vi "GUI.vi"(8 "error in (no error)":errorcluster) -> (0 "error out":errorcluster)   [LabVIEW 2020]
uses:
  CTLs/playback status.ctl
  FGVs/FGVstates.ctl
  CTLs/GUI_states.ctl
  CTLs/ButtonRefs.ctl
  FGVs/AppStates.ctl
panel:
  in  "Skip Forward Button":bool
  in  "Skip Back Button":bool
  out "Playback status":T1
  in  "Playlist":i32(listbox)
  out "Right Channel":dbl[](graph)
  out "Left Channel":dbl[](graph)
  in  "Pause Button":bool
  in  "Stop Button":bool
  in  "Play Button":bool
  in  "Playback Timeline":i32(slide) scale=0.0..11305728.0
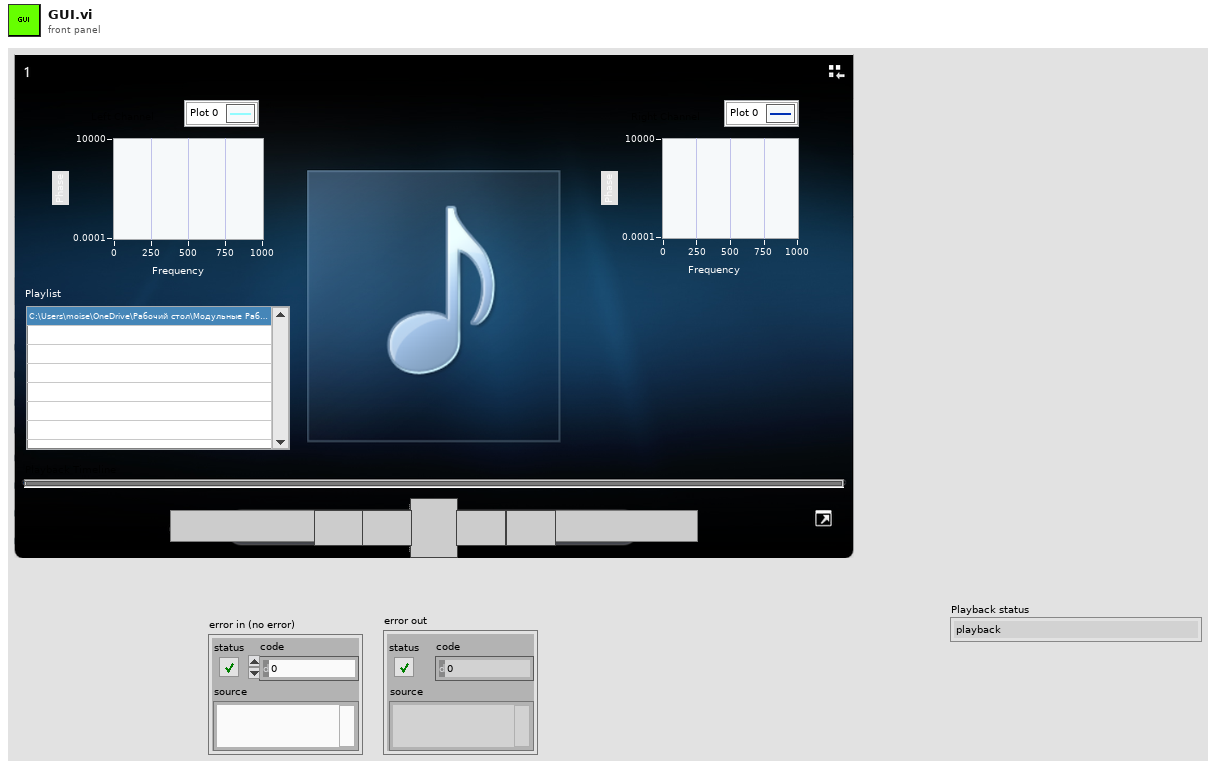
[diagram p1: front panel]
types:
  T1 = typedef "playback status.ctl" = enum16{"playback", "pause", "stop"}
  T2 = typedef "ButtonRefs.ctl" = cluster{"Button_play":refnum<vi>, "Button_pause":refnum<vi>, "Button_stop":refnum<vi>, "Playlist":refnum<vi>, "Playback status":refnum<vi>, "Playback Timeline":refnum<vi>, "Right Channel":refnum<vi>, "Left Channel":refnum<vi>, "Skip Forward Button":refnum<vi>, "Skip Back Button":refnum<vi>}
  T3 = typedef "GUI_states.ctl" = enum16{"Init Controls", "Prepare View Controls", "Idle"}
  T4 = typedef "FGVstates.ctl" = enum16{"Init", "Set", "Get", "De-Init"}
  T5 = typedef "data_exchange_fgv.ctl" = cluster{"queue states":refnum<queue>, "audio data":refnum<queue>, "error queue":refnum<queue>}
  T6 = typedef "AppStates.ctl" = enum16{"Init", "Scan Music Dir", "Idle", "Playback", "Enqueue samples", "Pause playback", "Stop playback", "Exit"}
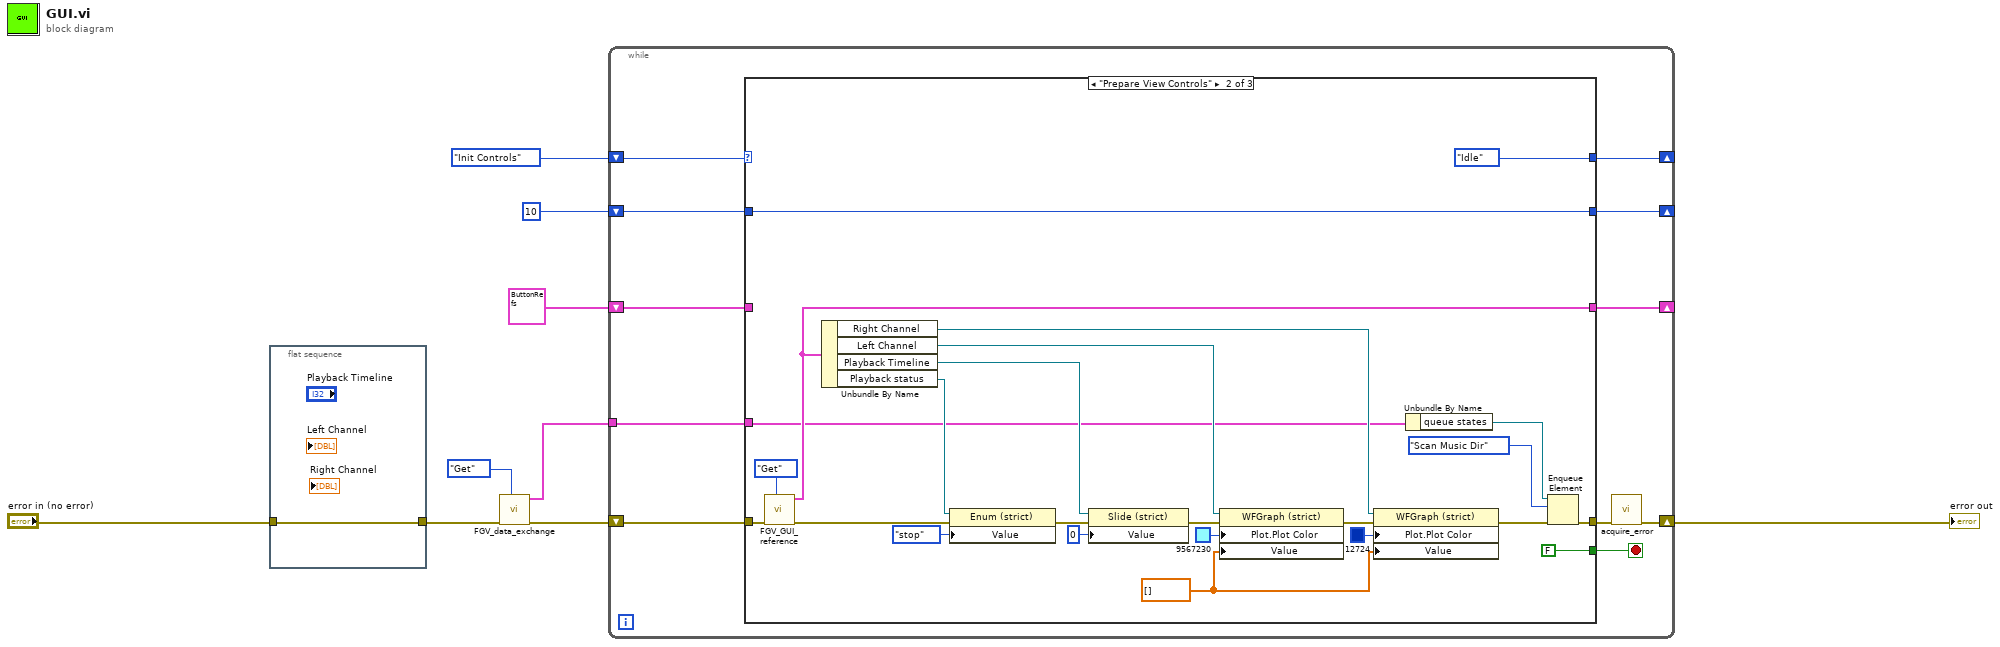
[diagram p0: block diagram]
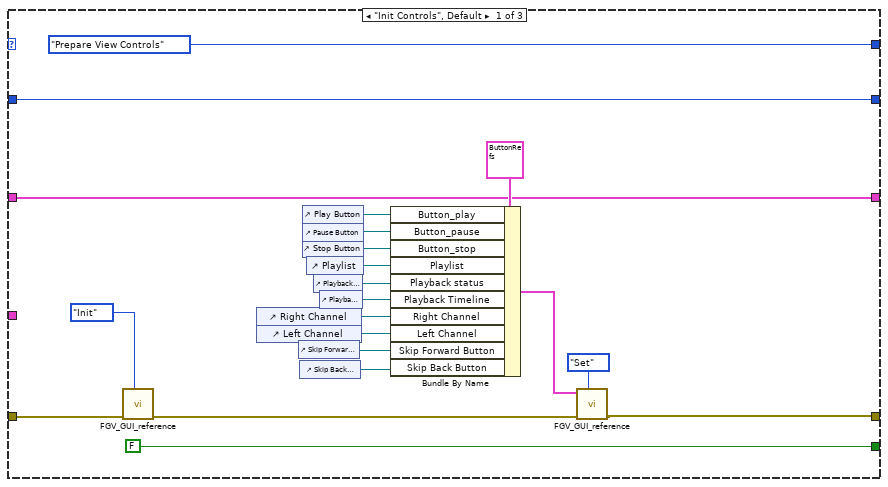
[diagram p2: hidden frame]
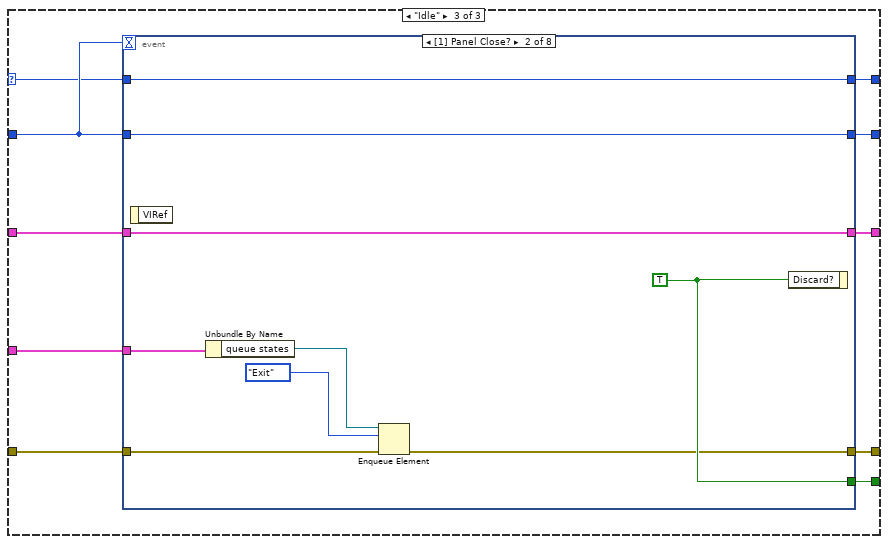
[diagram p3: hidden frame]
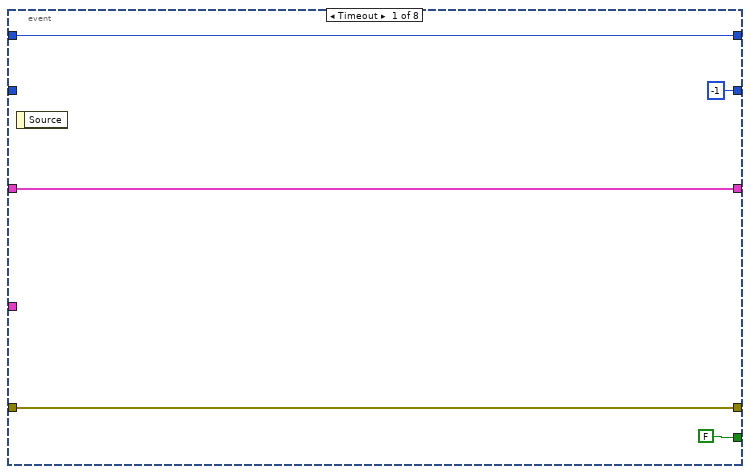
[diagram p4: hidden frame]
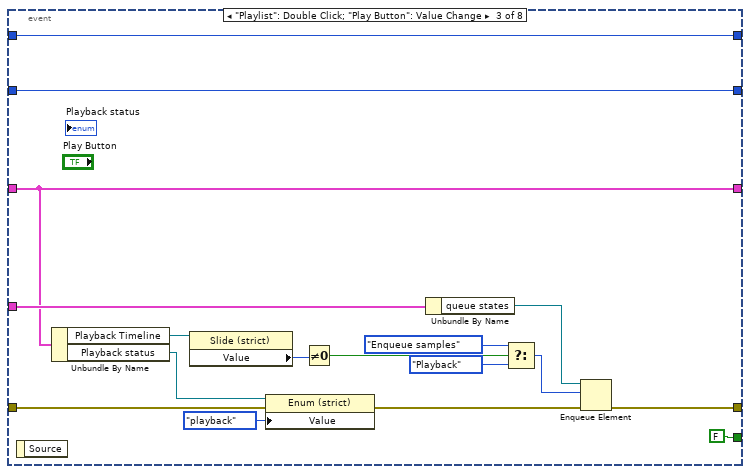
[diagram p5: hidden frame]
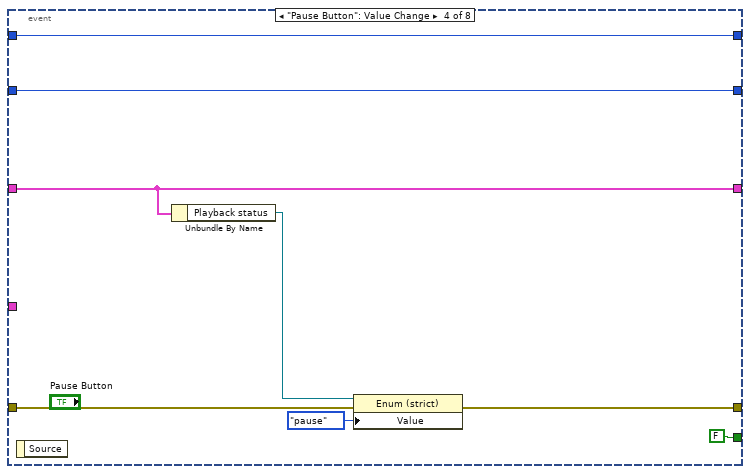
[diagram p6: hidden frame]
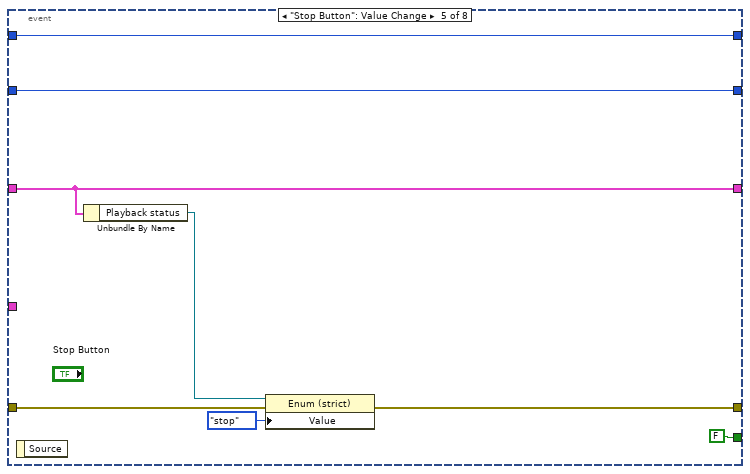
[diagram p7: hidden frame]
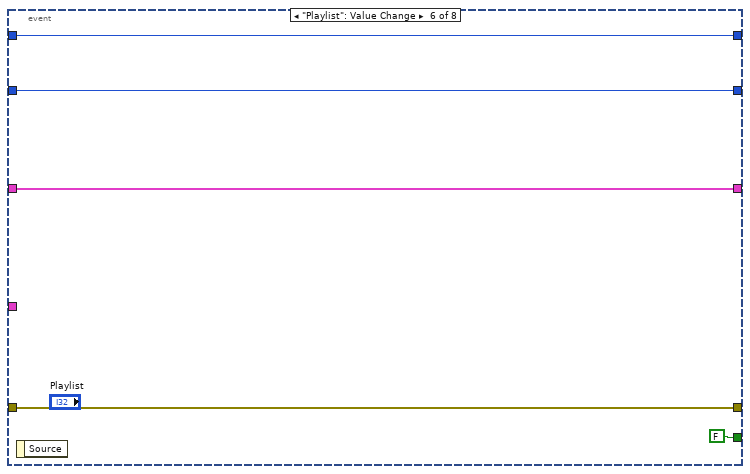
[diagram p8: hidden frame]
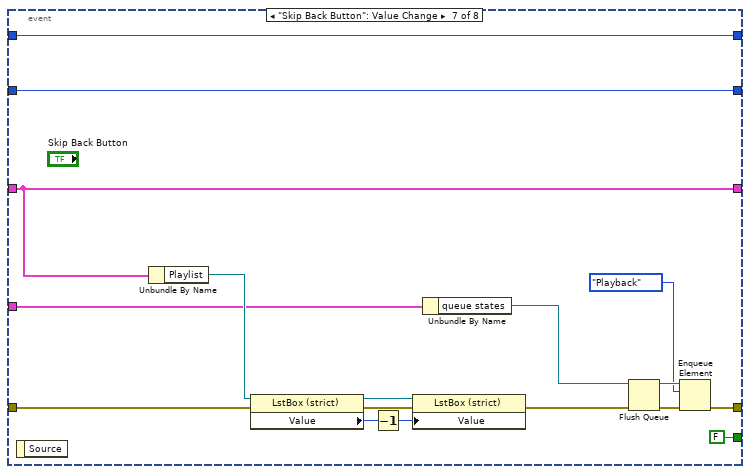
[diagram p9: hidden frame]
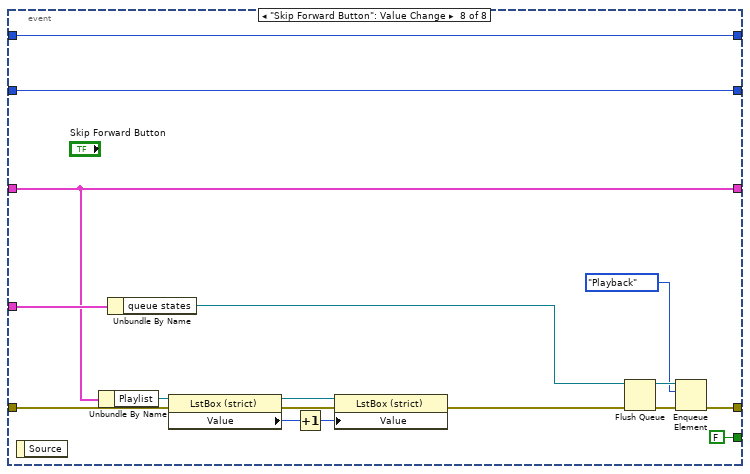
[diagram p10: hidden frame]
diagram:
  n1 = flat-sequence {
    tunnel: "error in (no error)" -> [w10]
    tunnel: [w10] -> w3
    frame #0 {
    }
  }
  n2 = call "FGV_data_exchange.vi"("FGV states"=FGVstates."Get", "error in (no error)"=w3) -> ("error out"=w5:errorcluster, "main_cycle_queue"=w7:T5)  [unwired: 8 in]
  n3 = while {
    shift-right: [w11] -> w9
    shift-left: w5 -> [w21]
    shift-right: [w19] -> _
    shift-left: 10 -> [w17]
    tunnel: w7 -> [w18]
    shift-right: [w16] -> _
    shift-left: T2 {"Button_play"=refnum, "Button_pause"=refnum, "Button_stop"=refnum, "Playlist"=refnum, "Playback status"=refnum, "Playback Timeline"=refnum, "Right Channel"=refnum, "Left Channel"=refnum, "Skip Forward Button"=refnum, "Skip Back Button"=refnum} ("Button refs Out") -> [w15]
    shift-right: [w13] -> _
    shift-left: GUI_states."Init Controls" -> [w14]
    stop <- w20 stop-if-true
    n4 = case shown="\"Prepare View Controls\"" w14 {
      selector: w14 -> [_ _ w68]
      tunnel: w21 -> [w26 w64 w76]
      tunnel: [w24 w44 w75] -> w12
      tunnel: [FALSE ("Discard?") FALSE ("Discard?") w74] -> w20
      tunnel: [w29 w48 w73] -> w19
      tunnel: w18 -> [_ w43 w72]
      tunnel: w17 -> [w29 w48 w71]
      tunnel: [w28 w63 w70] -> w16
      tunnel: w15 -> [w28 _ w69]
      tunnel: [GUI_states."Prepare View Controls" GUI_states."Idle" w67] -> w13
      frame "Init Controls", Default {
        n5 = call "FGV_GUI_reference.vi"("FGV states"=FGVstates."Init", "error in (no error)"=w26) -> ("error out"=w25:errorcluster)  [unwired: 8 in, 1 out]
        n6 = control-ref of="Right Channel"() -> (w36:refnum<vi>)
        n7 = control-ref of="Left Channel"() -> (w35:refnum<vi>)
        n8 = control-ref of="Skip Forward Button"() -> (w23:refnum<vi>)
        n9 = control-ref of="Skip Back Button"() -> (w22:refnum<vi>)
        n10 = control-ref of="Play Button"() -> (w42:refnum<vi>)
        n11 = control-ref of="Pause Button"() -> (w41:refnum<vi>)
        n12 = control-ref of="Stop Button"() -> (w40:refnum<vi>)
        n13 = control-ref of="Playlist"() -> (w39:refnum<vi>)
        n14 = control-ref of="Playback status"() -> (w38:refnum<vi>)
        n15 = control-ref of="Playback Timeline"() -> (w37:refnum<vi>)
        n16 = Bundle By Name(cluster=T2 {"Button_play"=refnum, "Button_pause"=refnum, "Button_stop"=refnum, "Playlist"=refnum, "Playback status"=refnum, "Playback Timeline"=refnum, "Right Channel"=refnum, "Left Channel"=refnum, "Skip Forward Button"=refnum, "Skip Back Button"=refnum} ("Button refs In"), "Button_play"=w42, "Button_pause"=w41, "Button_stop"=w40, "Playlist"=w39, "Playback status"=w38, "Playback Timeline"=w37, "Right Channel"=w36, "Left Channel"=w35, "Skip Forward Button"=w23, "Skip Back Button"=w22) -> (w30:T2)
        n17 = call "FGV_GUI_reference.vi"("FGV states"=FGVstates."Set", "error in (no error)"=w25, "Button refs In"=w30) -> ("error out"=w24:errorcluster)  [unwired: 7 in, 1 out]
      }
      frame "Prepare View Controls" {
        w50 = dbl[] [] ("Value")
        n18 = call "FGV_GUI_reference.vi"("FGV states"=FGVstates."Get", "error in (no error)"=w64) -> ("error out"=w62:errorcluster, "Button refs Out"=w63:T2)  [unwired: 8 in]
        n19 = Unbundle By Name(w63) -> ("Right Channel"=w51:refnum<vi>, "Left Channel"=w56:refnum<vi>, "Playback Timeline"=w58:refnum<vi>, "Playback status"=w61:refnum<vi>)
        n20 = property class="Enum (strict)"(reference=w61, error in=w62, "Value"=playback_status."stop") -> (error out=w59:errorcluster)  [unwired: 1 out]
        n21 = property class="Slide (strict)"(reference=w58, error in=w59, "Value"=0) -> (error out=w53:errorcluster)  [unwired: 1 out]
        n22 = property class="WFGraph (strict)"(reference=w56, error in=w53, "Plot.Plot Color"=u32 9567230, "Value"=w50) -> (error out=w54:errorcluster)  [unwired: 1 out]
        n23 = property class="WFGraph (strict)"(reference=w51, error in=w54, "Plot.Plot Color"=u32 12724, "Value"=w50) -> (error out=w45:errorcluster)  [unwired: 1 out]
        n24 = Unbundle By Name(w43) -> ("queue states"=w47:refnum<queue>)
        n25 = Enqueue Element(queue=w47, element=AppStates."Scan Music Dir", error in (no error)=w45) -> (error out=w44:errorcluster)  [unwired: 1 in, 2 out]
      }
      frame "Idle" {
        n26 = event shown="[1] Panel Close?" {
          selector: _ -> [_ _ _ _ _ _ _ _]
          dyn-events: _ -> [_ _ _ _ _ _ _ _]
          timeout: w71 -> [_ _ _ _ _ _ _ _]
          tunnel: w76 -> [w77 w87 w102 w112 w120 w128 w132 w150]
          tunnel: [w77 w85 w104 w111 w119 w128 w131 w158] -> w75
          tunnel: [FALSE w90 FALSE ("Discard?") FALSE ("Discard?") FALSE ("Discard?") FALSE ("Discard?") FALSE ("Discard?") FALSE ("Discard?")] -> w74
          tunnel: w71 -> [_ w89 w107 w114 w122 w126 w145 w162]
          tunnel: [-1 w89 w107 w114 w122 w126 w145 w162] -> w73
          tunnel: w72 -> [_ w88 w106 _ _ _ w130 w155]
          tunnel: [w78 w83 w93 w109 w117 w125 w129 w154] -> w70
          tunnel: w69 -> [w78 w83 w93 w109 w117 w125 w129 w154]
          tunnel: w68 -> [w79 w82 w94 w110 w118 w124 w144 w161]
          tunnel: [w79 w82 w94 w110 w118 w124 w144 w161] -> w67
          event Timeout {
            n27 = event-data() -> ()  [unwired: 1 in, 1 out]
          }
          event Panel Close? {
            w90 = TRUE ("Discard?")
            n28 = event-data() -> ()  [unwired: 1 in, 1 out]
            n29 = Unbundle By Name(w88) -> ("queue states"=w86:refnum<queue>)
            n30 = Enqueue Element(queue=w86, element=AppStates."Exit", error in (no error)=w87) -> (error out=w85:errorcluster)  [unwired: 1 in, 2 out]
            n31 = event-data("Discard?"=w90) -> ()  [unwired: 1 in, 1 out]
          }
          event "Playlist": Double Click; "Play Button": Value Change {
            n32 = event-data() -> ()  [unwired: 1 in, 1 out]
            n33 = Unbundle By Name(w93) -> ("Playback Timeline"=w92:refnum<vi>, "Playback status"=w91:refnum<vi>)
            n34 = property class="Slide (strict)"(reference=w92) -> ("Value"=w99:i32)  [unwired: 1 in, 2 out]
            n35 = property class="Enum (strict)"(reference=w91, error in=w102, "Value"=playback_status."playback") -> (error out=w100:errorcluster)  [unwired: 1 out]
            n36 = Not Equal To 0?(x=w99) -> (x != 0?=w98:bool)
            n37 = Unbundle By Name(w106) -> ("queue states"=w105:refnum<queue>)
            n38 = Select(t=AppStates."Enqueue samples" ("element"), s=w98, f=AppStates."Playback" ("element")) -> (s? t:f=w95:T6)
            n39 = Enqueue Element(queue=w105, element=w95, error in (no error)=w100) -> (error out=w104:errorcluster)  [unwired: 1 in, 2 out]
          }
          event "Pause Button": Value Change {
            n40 = event-data() -> ()  [unwired: 1 in, 1 out]
            n41 = Unbundle By Name(w109) -> ("Playback status"=w108:refnum<vi>)
            n42 = property class="Enum (strict)"(reference=w108, error in=w112, "Value"=playback_status."pause") -> (error out=w111:errorcluster)  [unwired: 1 out]
          }
          event "Stop Button": Value Change {
            n43 = event-data() -> ()  [unwired: 1 in, 1 out]
            n44 = Unbundle By Name(w117) -> ("Playback status"=w116:refnum<vi>)
            n45 = property class="Enum (strict)"(reference=w116, error in=w120, "Value"=playback_status."stop") -> (error out=w119:errorcluster)  [unwired: 1 out]
          }
          event "Playlist": Value Change {
            n46 = event-data() -> ()  [unwired: 1 in, 1 out]
          }
          event "Skip Back Button": Value Change {
            n47 = event-data() -> ()  [unwired: 1 in, 1 out]
            n48 = Unbundle By Name(w129) -> ("Playlist"=w138:refnum<vi>)
            n49 = property class="LstBox (strict)"(reference=w138, error in=w132) -> (reference out=w133:refnum<vi>, error out=w135:errorcluster, "Value"=w137:i32)
            n50 = Decrement(x=w137) -> (x-1=w136:i32)
            n51 = property class="LstBox (strict)"(reference=w133, error in=w135, "Value"=w136) -> (error out=w134:errorcluster)  [unwired: 1 out]
            n52 = Unbundle By Name(w130) -> ("queue states"=w140:refnum<queue>)
            n53 = Flush Queue(queue=w140, error in (no error)=w134) -> (queue out=w142:refnum<queue>, error out=w141:errorcluster)  [unwired: 1 out]
            n54 = Enqueue Element(queue=w142, element=AppStates."Playback", error in (no error)=w141) -> (error out=w131:errorcluster)  [unwired: 1 in, 2 out]
          }
          event "Skip Forward Button": Value Change {
            n55 = event-data() -> ()  [unwired: 1 in, 1 out]
            n56 = Unbundle By Name(w154) -> ("Playlist"=w153:refnum<vi>)
            n57 = Unbundle By Name(w155) -> ("queue states"=w157:refnum<queue>)
            n58 = property class="LstBox (strict)"(reference=w153, error in=w150) -> (reference out=w146:refnum<vi>, error out=w149:errorcluster, "Value"=w152:i32)
            n59 = Increment(x=w152) -> (x+1=w151:i32)
            n60 = property class="LstBox (strict)"(reference=w146, error in=w149, "Value"=w151) -> (error out=w148:errorcluster)  [unwired: 1 out]
            n61 = Flush Queue(queue=w157, error in (no error)=w148) -> (queue out=w160:refnum<queue>, error out=w159:errorcluster)  [unwired: 1 out]
            n62 = Enqueue Element(queue=w160, element=AppStates."Playback", error in (no error)=w159) -> (error out=w158:errorcluster)  [unwired: 1 in, 2 out]
          }
        }
      }
    }
    n63 = call "acquire_error.vi"("error in (no error)"=w12) -> ("error out"=w11:errorcluster)  [unwired: 10 in]
  }
  "error out" <- w9
